vi "SetUpE4418B.vi"(2 "error in (no error)":errorcluster) -> (0 "error out":errorcluster)   [LabVIEW 2009]
doc: "Set up defaults for E4418B average power measurements at TOF transmitter\nwhich may disable automatic parameter selection for optimum Tx pwr measurements.\nVarious special \"manual\" modes may be used to measure power consistently \nfrom signal generator, noise generators, or pulsed transmitters.\nMay sometimes use triggered measurements to try to improve stability on avg Tx pulse power."
panel:
  in  "SCPI commands":string="*cls\nSYST:PRES\nSENS:FREQ 2850MHz\nSENS:AVER:SDET OFF\nSENS:AVER:COUNT  64\nSENS:AVER:COUNT:AUTO OFF\nSENS:AVER:STATE ON\nDISP:WIND1:RES 3\n\n"
  # "Set up defaults for E4418B average power measurements  at TOF transmitter\nwhich may disable automatic parameter selection for optimum Tx pwr measurements.\nVarious special \"manual\"  modes may be used to measure power consistently \nfrom  signal generator, noise generators, or pulsed transmitters. May sometimes use triggered measurements to try to improve stability on avg Tx pulse power."
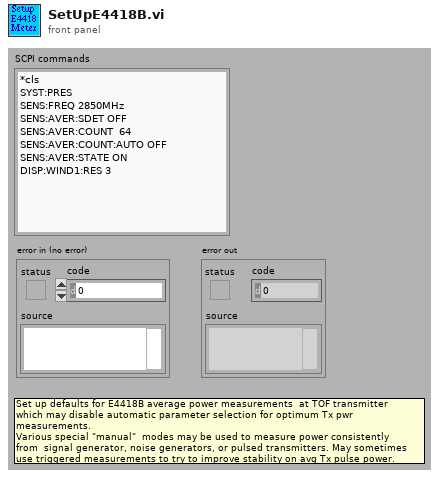
[diagram p1: front panel]
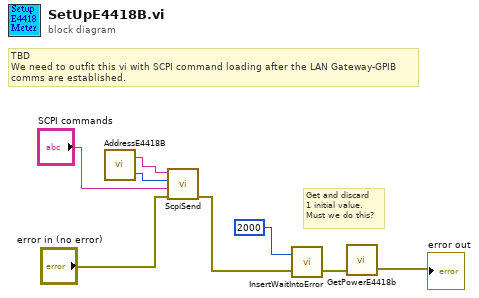
[diagram p0: block diagram]
diagram:
  # "Get and discard\n1 initial value.\nMust we do this?"
  # "TBD\nWe need to outfit this vi with SCPI command loading after the LAN Gateway-GPIB comms are established."
  n1 = call "AddressE4418B.vi"() -> ("Port"=w2:i32, "IP address"=w1:string)  [unwired: 2 in]
  n2 = call "ScpiSend.vi"("error in (no error)"="error in (no error)", "Command"="SCPI commands", "TCP port"=w2, "IP Address"=w1) -> ("error out"=w5:errorcluster)  [unwired: 7 in]
  n3 = call "InsertWaitIntoError.vi"("error in (no error)"=w5, "Wait (msecs)"=2000 ("PauseBeforeFirstReading")) -> ("error out"=w8:errorcluster)  [unwired: 1 in]
  n4 = call "GetPowerE4418b.vi"("error in (no error)"=w8) -> ("Error out"=→"error out":errorcluster)  [unwired: 1 in, 1 out]
